vi "rqcAlice Attenuator Control.vi"() -> ()   [LabVIEW 2018]
uses:
  <vilib>/FPGAPlugInAG/PCIe-7820R/niLvFpga_Open_PCIe-7820R.vi
  <vilib>/rvi/interface/common/dynamic/niFpgaDynamicAddResources.vi
  <vilib>/FPGAPlugInAG/Dynamic/niLvFpga_Close_Dynamic.vi
  <vilib>/rvi/interface/nirviOpenFPGA/nirviOpenFPGA.xnode
  FPGA Bitfiles/rqcAlice FPGA (7820R) v 2.3.0.lvbitx
  <vilib>/rvi/interface/nirviCloseFPGA/nirviCloseFPGA.xnode
panel:
  in  "stop":bool
  in  "Attenuation, dB":fxp<+,7,6>=10.0
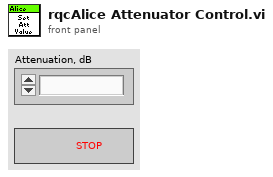
[diagram p1: front panel]
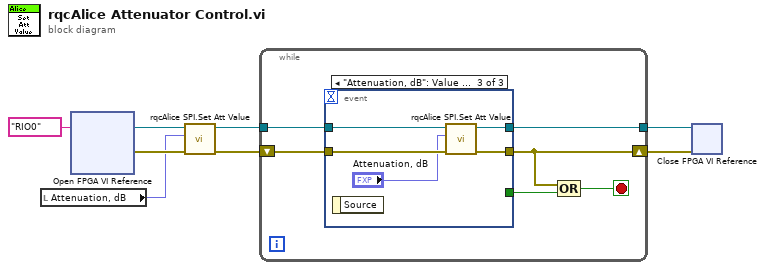
[diagram p0: block diagram]
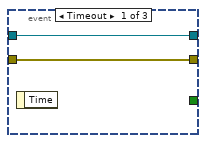
[diagram p2: hidden frame]
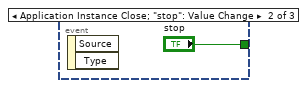
[diagram p3: hidden frame]
diagram:
  n1 = local read "Attenuation, dB"() -> (w3:fxp<+,7,6>)
  n2 = xnode "Open FPGA VI Reference"("resource name"=tag "RIO0") -> ("FPGA VI Reference Out"=w7:refnum<k20>, "error out"=w5:errorcluster)  [unwired: 1 in]
  n3 = call "rqcAlice SPI.Set Att Value.vi"("error in"=w5, "Attenuation, dB"=w3, "Alice FPGA Reference In"=w7) -> ("error out"=w4:errorcluster, "Alice FPGA Reference Out"=w6:refnum<k20>)  [unwired: 7 in]
  n4 = while {
    tunnel: w6 -> [w14]
    tunnel: [w12] -> w1
    shift-right: [w10] -> w2
    shift-left: w4 -> [w13]
    stop <- w11 stop-if-true
    n5 = event shown="[2] \"Attenuation, dB\": Value Change" {
      selector: _ -> [_ _ _]
      dyn-events: _ -> [_ _ _]
      timeout: _ -> [_ _ _]
      tunnel: w14 -> [w15 _ w22]
      tunnel: w13 -> [w16 _ w21]
      tunnel: [w16 _ w19] -> w10
      tunnel: [w15 _ w18] -> w12
      tunnel: [_ "stop" _] -> w9
      event Timeout {
        n6 = event-data() -> ()  [unwired: 1 in, 1 out]
      }
      event Application Instance Close; "stop": Value Change {
        n7 = event-data() -> ()  [unwired: 1 in, 2 out]
      }
      event "Attenuation, dB": Value Change {
        n8 = event-data() -> ()  [unwired: 1 in, 1 out]
        n9 = call "rqcAlice SPI.Set Att Value.vi"("error in"=w21, "Attenuation, dB"="Attenuation, dB", "Alice FPGA Reference In"=w22) -> ("error out"=w19:errorcluster, "Alice FPGA Reference Out"=w18:refnum<k20>)  [unwired: 7 in]
      }
    }
    n10 = Compound Arithmetic op=OR(w10, w9) -> (w11:bool)
  }
  n11 = xnode "Close FPGA VI Reference"("FPGA VI Reference In"=w1, "error in"=w2) -> ()  [unwired: 1 out]
